vi "Mandelbrot_CuLab.vi"(7 "Max_iter":i32=4000, 8 "Zoom":dbl=5e-11, 9 "y":dbl=0.13182590420533, 10 "x":dbl=-0.743643887037151, 11 "Resolution":i32=1000) -> (0 "Exec Time":dbl=3.6367448000000877, 3 "Mandelbrot Graph":i16[][](graph))   [LabVIEW 2020]
uses:
  <vilib>/Ngene/CuLab - GPU Accelerated Toolkit/Toolkit/Low_Level/Tensor_Classes/T_Children/T2D/Controls/T2D_Dims.ctl
  <vilib>/Ngene/CuLab - GPU Accelerated Toolkit/Toolkit/Low_Level/GPU_Wrapper/culab_comparison/Controls/culab_comp_mode_2in.ctl
  <vilib>/Ngene/CuLab - GPU Accelerated Toolkit/Toolkit/Low_Level/GPU_Wrapper/culab_comparison/Controls/culab_bool_neg_inputs.ctl
  <vilib>/Ngene/CuLab - GPU Accelerated Toolkit/Toolkit/Low_Level/GPU_Wrapper/culab_comparison/Controls/culab_bool_op_2in.ctl
  250ad98c-c819-4240-bb72-613057cdb05b.vi
  <vilib>/Ngene/CuLab - GPU Accelerated Toolkit/Toolkit/Low_Level/Tensor_Classes/T_Children/T2D/T2D_Children/T2D_I16/Pull.vi
  8fc4144a-0758-458b-88ac-401a6681cd74.vi
  <vilib>/Analysis/1siggen.llb/Ramp Pattern by Samples.vi
  <vilib>/Utility/High Resolution Relative Seconds.vi
  <vilib>/Ngene/CuLab - GPU Accelerated Toolkit/Toolkit/Low_Level/GPU_Wrapper/cudart/Memory/PULL/2D/cudart_PULL_Data(I16_2D).vi
  <vilib>/Ngene/CuLab - GPU Accelerated Toolkit/Toolkit/Low_Level/Tensor_Classes/T_Children/T2D/T2D_Children/T2D_CDB/T2D_CDB.lvclass
  C:/Program Files/National Instruments/LabVIEW 2020/vi.lib/Ngene/CuLab - GPU Accelerated Toolkit/Toolkit/Low_Level/Tensor_Classes/T_Children/T2D/T2D.lvclass
  <vilib>/Ngene/CuLab - GPU Accelerated Toolkit/Toolkit/Low_Level/Tensor_Classes/T_Children/T2D/T2D_Children/T2D_U8/T2D_U8.lvclass
  <vilib>/Ngene/CuLab - GPU Accelerated Toolkit/Toolkit/Low_Level/Tensor_Classes/T_Children/T2D/T2D_Children/T2D_I16/T2D_I16.lvclass
  C:/Program Files/National Instruments/LabVIEW 2020/vi.lib/Ngene/CuLab - GPU Accelerated Toolkit/Toolkit/Low_Level/Tensor_Classes/Tensor.lvclass
  <vilib>/Ngene/CuLab - GPU Accelerated Toolkit/Toolkit/Low_Level/Tensor_Classes/T_Children/T2D/T2D_Children/T2D_CDB/Create_Push.vi
  <vilib>/Ngene/CuLab - GPU Accelerated Toolkit/Toolkit/API/Array/Initialize Array/T2D/CU_Initialize Array_T2D_I16.vi
  <vilib>/Ngene/CuLab - GPU Accelerated Toolkit/Toolkit/API/Array/Initialize Array/T2D/CU_Initialize Array_T2D_U8.vi
  <vilib>/Ngene/CuLab - GPU Accelerated Toolkit/Toolkit/API/Numeric/Multiply/T2D/CU_MultiplyC_T2D_CDB.vi
  <vilib>/Ngene/CuLab - GPU Accelerated Toolkit/Toolkit/API/Numeric/Square/T2D/CU_Square_T2D_CDB.vi
  <vilib>/Ngene/CuLab - GPU Accelerated Toolkit/Toolkit/API/Numeric/Add/T2D/CU_Add_T2D_CDB.vi
  <vilib>/Ngene/CuLab - GPU Accelerated Toolkit/Toolkit/API/Numeric/Conversion  (API)/CSG/CU_To_CSG_T2D.vi
  <vilib>/Ngene/CuLab - GPU Accelerated Toolkit/Toolkit/API/Numeric/Absolute/T2D/CU_Absolute_T2D_CSG.vi
  <vilib>/Ngene/CuLab - GPU Accelerated Toolkit/Toolkit/API/Comparison/Compare_2_Inputs/T2D/CU_Compare_2InC_T2D_SGL.vi
  <vilib>/Ngene/CuLab - GPU Accelerated Toolkit/Toolkit/API/Boolean/Boolean_2in/T2D/CU_Boolean_2In_T2D_U8.vi
  <vilib>/Ngene/CuLab - GPU Accelerated Toolkit/Toolkit/API/Numeric/Conversion  (API)/I16/CU_To_I16_T2D.vi
  <vilib>/Ngene/CuLab - GPU Accelerated Toolkit/Toolkit/API/Numeric/Multiply/T2D/CU_MultiplyC_T2D_I16.vi
  <vilib>/Ngene/CuLab - GPU Accelerated Toolkit/Toolkit/API/Numeric/Add/T2D/CU_Add_T2D_I16.vi
  <vilib>/Ngene/CuLab - GPU Accelerated Toolkit/Toolkit/Low_Level/Checkers/Check_Tensor_Ref.vi
  <vilib>/Ngene/CuLab - GPU Accelerated Toolkit/Toolkit/Low_Level/Tensor_Classes/Property/Get_Mem_Desc.vi
  <vilib>/Ngene/CuLab - GPU Accelerated Toolkit/Toolkit/Low_Level/Tensor_Classes/T_Children/T2D/Property/Get_Dims.vi
  <vilib>/Ngene/CuLab - GPU Accelerated Toolkit/Toolkit/Low_Level/GPU_Wrapper/cudart/Memory/Utils/cudart_get_type_size(inBytes).vi
  <vilib>/Ngene/CuLab - GPU Accelerated Toolkit/Toolkit/Low_Level/GPU_Wrapper/cudart/cudart_get_Error_String.vi
  <vilib>/Analysis/NI_AALBase.lvlib
  <vilib>/Ngene/CuLab - GPU Accelerated Toolkit/Toolkit/CuLab.lvlib
  C:/Program Files/National Instruments/LabVIEW 2020/vi.lib/Ngene/CuLab - GPU Accelerated Toolkit/Toolkit/Low_Level/Tensor_Classes/T_Children/T2D/T2D_Children/T2D_CDB/T2D_CDB.lvclass
  C:/Program Files/National Instruments/LabVIEW 2020/vi.lib/Ngene/CuLab - GPU Accelerated Toolkit/Toolkit/Low_Level/Tensor_Classes/T_Children/T2D/T2D_Children/T2D_U8/T2D_U8.lvclass
panel:
  out "Iteration":i32=3999
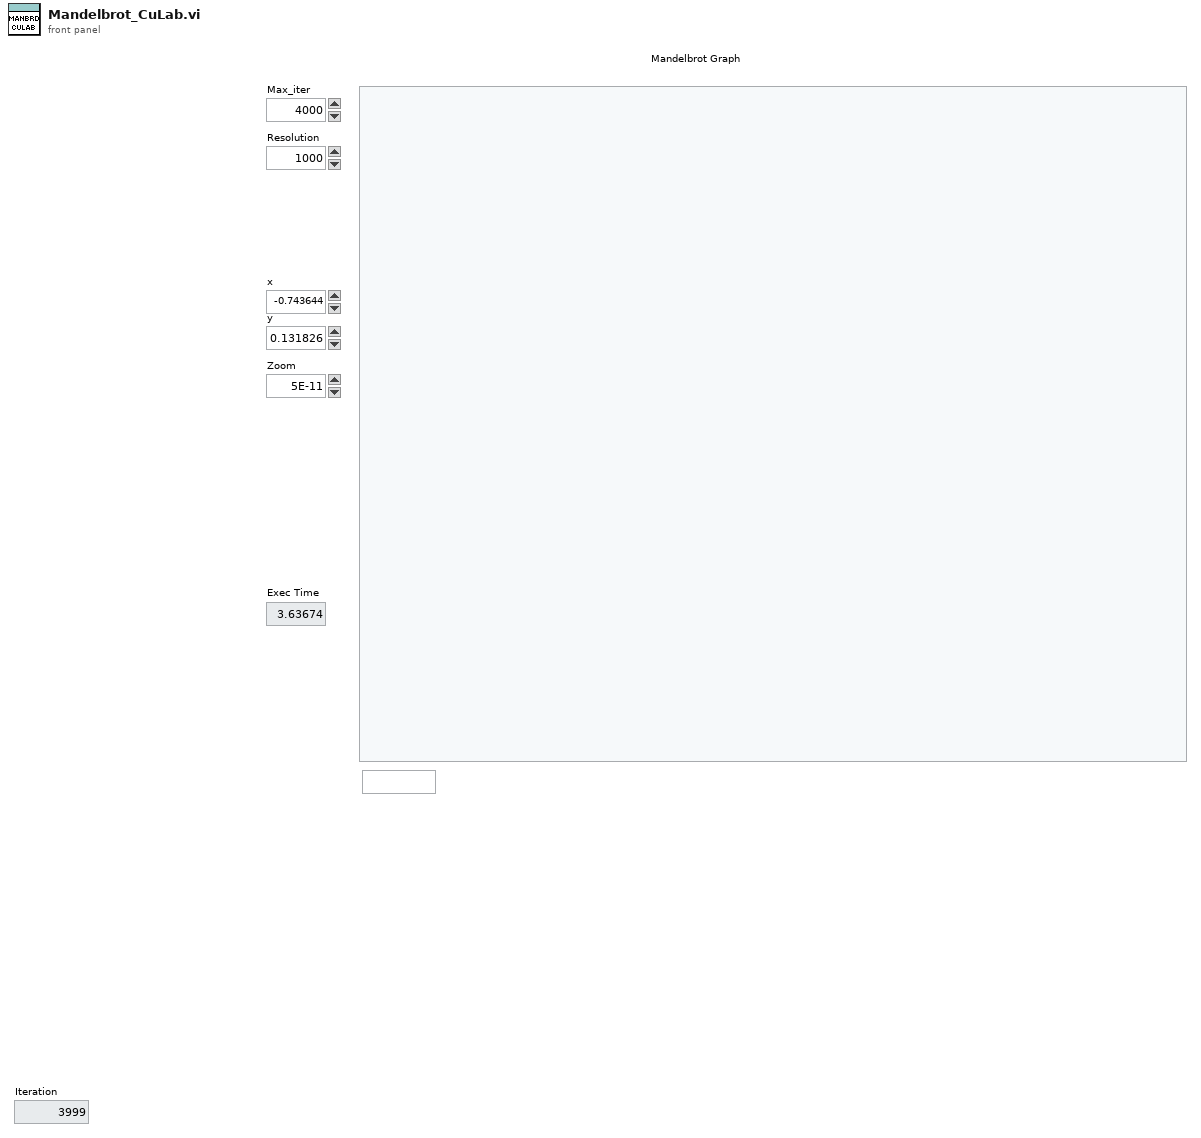
[diagram p1: front panel]
types:
  T1 = typedef "CuLab.lvlib/T2D_Dims.ctl" = cluster{"H":i32, "W":i32}
  T2 = typedef "CuLab.lvlib/culab_comp_mode_2in.ctl" = enum8{"Equal?", "Not Equal?", "Greater?", "Greater Or Equal?", "Less?", "Less Or Equal?"}
  T3 = typedef "CuLab.lvlib/culab_bool_neg_inputs.ctl" = enum32{"None", "First Input", "Second Input", "Both"}
  T4 = typedef "CuLab.lvlib/culab_bool_op_2in.ctl" = enum32{"AND", "OR", "XOR", "NAND", "NOR", "XNOR", "Select X", "Select Y"}
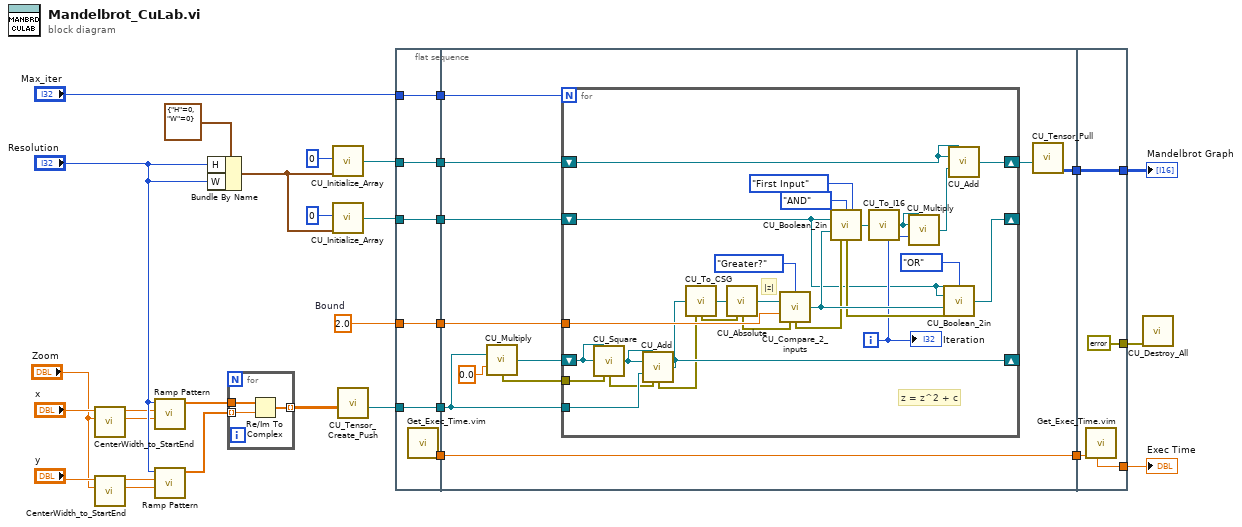
[diagram p0: block diagram]
diagram:
  w4 = sgl 2.0  # Bound
  n1 = call "CenterWidth_to_StartEnd.vi"("width"="Zoom", "Center"="x") -> ("Start"=w17:dbl, "End"=w18:dbl)  [unwired: 8 in]
  n2 = call "CenterWidth_to_StartEnd.vi"("width"="Zoom", "Center"="y") -> ("Start"=w13:dbl, "End"=w14:dbl)  [unwired: 8 in]
  n3 = call-poly <vilib>:"Ramp Pattern.vi"("start"=w17, "end"=w18, "samples"="Resolution") -> ("Ramp Pattern"=w16:dbl[])  [unwired: 7 in, 1 out]
  n4 = call-poly <vilib>:"Ramp Pattern.vi"("start"=w13, "end"=w14, "samples"="Resolution") -> ("Ramp Pattern"=w15:dbl[])  [unwired: 7 in, 1 out]
  n5 = Bundle By Name(cluster=T1 {"H"=0, "W"=0} ("dimension sizes"), "H"="Resolution", "W"="Resolution") -> (w5:T1)
  n6 = for {
    tunnel: w15 -> [w33] mode=indexing
    tunnel: w16 -> [w34]
    tunnel: [w32] -> w12 mode=indexing
    n7 = Re/Im To Complex(1:w33, 2:w34) -> (0:w32:cdb[])
  }
  n8 = call-poly <vilib>:"CU_Initialize_Array.vi"("element"=i16 0, "dimension sizes"=w5) -> ("initialized Tensor"=w8:refnum<class "T2D_I16.lvclass">)  [unwired: 12 in, 1 out]
  n9 = call-poly <vilib>:"CU_Initialize_Array.vi"("element"=i16 0, "dimension sizes"=w5) -> ("initialized Tensor"=w6:refnum<class "T2D_U8.lvclass">)  [unwired: 12 in, 1 out]
  n10 = call-poly <vilib>:"CU_Tensor_Create_Push.vi"("CPU_Data_2D_CDB"=w12) -> ("T2D_CDB out"=w11:refnum<class "T2D_CDB.lvclass">)  [unwired: 9 in, 1 out]
  n11 = flat-sequence {
    tunnel: w11 -> [w38]
    tunnel: w6 -> [w39]
    tunnel: "Max_iter" -> [w40]
    tunnel: [w40] -> w26
    tunnel: [w39] -> w25
    tunnel: [w38] -> w24
    tunnel: [w37] -> w23
    tunnel: [w36] -> w22
    tunnel: w8 -> [w36]
    tunnel: [w35] -> w21
    tunnel: w4 -> [w35]
    tunnel: w26 -> [w51]
    tunnel: w25 -> [w50]
    tunnel: w24 -> [w48]
    tunnel: [w43] -> w20
    tunnel: w23 -> [w43]
    tunnel: w22 -> [w49]
    tunnel: [w44] -> w19
    tunnel: w21 -> [w42]
    tunnel: w20 -> [w82]
    tunnel: [w81] -> w2
    tunnel: [errorcluster {"status"=FALSE, "code"=0, "source"=""} ("error out")] -> w3
    tunnel: [w80] -> w1
    tunnel: w19 -> [w80]
    frame #0 {
      n12 = call "Get_Exec_Time.vim"() -> ("T(n)"=w37:dbl)  [unwired: 7 in, 2 out]
    }
    frame #1 {
      n13 = call-poly <vilib>:"CU_Multiply.vi"("x"=w48, "y"=sgl 0.0 ("start")) -> ("Dest out"=w47:refnum<class "T2D_CDB.lvclass">, "error out"=w41:errorcluster)  [unwired: 12 in]
      n14 = for {
        N: w51 -> [_]
        shift-right: [w63] -> _
        shift-left: w47 -> [w64]
        tunnel: w48 -> [w75]
        shift-right: [w78] -> w45
        shift-left: w49 -> [w68]
        tunnel: w42 -> [w76]
        shift-right: [w77] -> _
        shift-left: w50 -> [w52]
        tunnel: w41 -> [w53]
        i -> [w65]
        # "|z|"
        # "z = z^2 + c"
        n15 = call-poly <vilib>:"CU_Square.vi"("Dest in"=w64, "x"=w64, "error in (no error)"=w53) -> ("Dest out"=w59:refnum<class "T2D_CDB.lvclass">, "error out"=w58:errorcluster)  [unwired: 11 in]
        n16 = call-poly <vilib>:"CU_Add.vi"("Dest in"=w59, "x"=w59, "y"=w75, "error in (no error)"=w58) -> ("Dest out"=w63:refnum<class "T2D_CDB.lvclass">, "error out"=w57:errorcluster)  [unwired: 10 in]
        n17 = call-poly <vilib>:"CU_To_CSG.vi"("Tensor in"=w63, "error in (no error)"=w57) -> ("Dest out"=w60:refnum<class "T2D_CSG.lvclass">, "error out"=w56:errorcluster)  [unwired: 12 in]
        n18 = call-poly <vilib>:"CU_Absolute.vi"("x"=w60, "error in (no error)"=w56) -> ("Dest out"=w62:refnum<class "T2D_SGL.lvclass">, "error out"=w55:errorcluster)  [unwired: 12 in]
        n19 = call-poly <vilib>:"CU_Compare_2_inputs.vi"("Comp Mode"=culab_comp_mode_2in."Greater?", "x"=w62, "y"=w76, "error in (no error)"=w55) -> ("Dest out"=w71:refnum<class "T2D_U8.lvclass">, "error out"=w54:errorcluster)  [unwired: 10 in]
        n20 = call-poly <vilib>:"CU_Boolean_2in.vi"("Bool Operation"=culab_bool_op_2in."AND", "Negate input/s?"=culab_bool_neg_inputs."First Input", "x"=w52, "y"=w71, "error in (no error)"=w54) -> ("Dest out"=w70:refnum<class "T2D_U8.lvclass">, "error out"=w66:errorcluster)  [unwired: 9 in]
        n21 = call-poly <vilib>:"CU_To_I16.vi"("Tensor in"=w70) -> ("Dest out"=w67:refnum<class "T2D_I16.lvclass">)  [unwired: 13 in, 1 out]
        n22 = call-poly <vilib>:"CU_Multiply.vi"("Dest in"=w67, "x"=w67, "y"=w65) -> ("Dest out"=w69:refnum<class "T2D_I16.lvclass">)  [unwired: 11 in, 1 out]
        n23 = call-poly <vilib>:"CU_Boolean_2in.vi"("Dest In"=w52, "Bool Operation"=culab_bool_op_2in."OR", "x"=w52, "y"=w71, "error in (no error)"=w66) -> ("Dest out"=w77:refnum<class "T2D_U8.lvclass">)  [unwired: 9 in, 1 out]
        n24 = call-poly <vilib>:"CU_Add.vi"("Dest in"=w68, "x"=w68, "y"=w69) -> ("Dest out"=w78:refnum<class "T2D_I16.lvclass">)  [unwired: 11 in, 1 out]
        "Iteration" <- w65
      }
      n25 = call-poly <vilib>:"CU_Tensor_Pull.vi"("T2D_I16 in"=w45) -> ("Dest out"=w44:i16[][])  [unwired: 8 in, 2 out]
    }
    frame #2 {
      n26 = call "Get_Exec_Time.vim"("T(n-1)"=w82) -> ("dT"=w81:dbl)  [unwired: 6 in, 2 out]
    }
  }
  n27 = call <vilib>:"CU_Destroy_All.vi"("error in"=w3) -> ()  [unwired: 10 in, 1 out]
  "Mandelbrot Graph" <- w1
  "Exec Time" <- w2
